vi "SPD.Update Lists.vi"(0 "SPD.Stand Ctrl in":T1 {"spdDeviceSession"."hidSPD.Controller"."HV_bias" format="%#_6p, V"; "spdDeviceSession"."hidSPD.Controller"."TSet" format="%#_6p, DegC"}, 11 "Error In":errorcluster, 12 "Temperature_List":refnum<vi>, 13 "Stb_code_List":refnum<vi>, 14 "HV_bias_List":refnum<vi>) -> (4 "SPD.Stand Ctrl out":T1 {"spdDeviceSession"."hidSPD.Controller"."HV_bias" format="%#_6p, V"; "spdDeviceSession"."hidSPD.Controller"."TSet" format="%#_6p, DegC"}, 15 "Error Out":errorcluster)   [LabVIEW 2018]
uses:
  typedefs/SPD.Stand Ctrl.ctl
  Instruments/SPD HID Interface/hidSPDLibForLabView/LibVIs/hidSPD Controls/hidSPD Device Session.ctl
  Instruments/SPD HID Interface/hidSPDLibForLabView/LibVIs/hidSPD Controls/hidSPD Controller.ctl
  Instruments/KC705 DevBoard/typedefs/DevB.Session.ctl
  Instruments/KeySight 53230A/typedefs/FreqC.Session.ctl
  Instruments/KeySight 8164B/KeySight 8164B LAN InstrLib/typedefs/KeySight 8164B control.ctl
  Instruments/LeCroy SDA830/typedefs/LeCroy.Session.ctl
  typedefs/SPD.Events.ctl
  <vilib>/Utility/config.llb/Config Data RefNum.ctl
  typedefs/SPD.Meas Result.ctl
  Instruments/SPD HID Interface/hidSPDLibForLabView/hidSPDLibForLabView.lvlib
  Instruments/KeySight 8164B/KeySight 8164B LAN InstrLib.lvlib
  <vilib>/Utility/config.llb/NI_LVConfig.lvlib
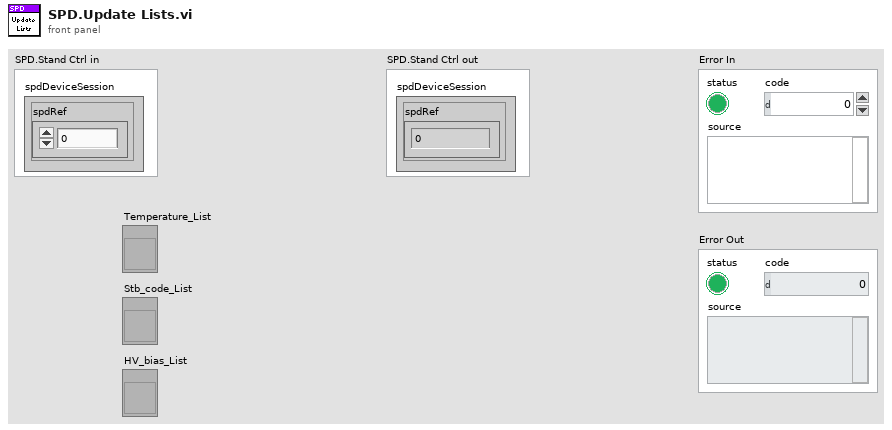
[diagram p1: front panel]
types:
  T1 = typedef "SPD.Stand Ctrl.ctl" = cluster{"spdDeviceSession":T2, "DevBSession":T4, "FreqCSession":T5, "8164BSession":T6, "LeCroySession":T7, "Events":T8, "configFile":T9, "SPD.Result":T10}
  T2 = typedef "hidSPDLibForLabView.lvlib/hidSPD Device Session.ctl" = cluster{"spdRef":u64, "connected":bool, "spdName":string, "hidSPD.Controller":T3}
  T3 = typedef "hidSPDLibForLabView.lvlib/hidSPD Controller.ctl" = cluster{"TSet":sgl, "HV_bias":sgl, "DDS_stb_code":u16}
  T4 = typedef "DevB.Session.ctl" = cluster{"DevBRef":refnum<visa-resource-name>, "connected":bool}
  T5 = typedef "FreqC.Session.ctl" = cluster{"FreqCRef":refnum<visa-resource-name>, "timeout":dbl, "Gate":dbl, "connected":bool}
  T6 = typedef "KeySight 8164B LAN InstrLib.lvlib/KeySight 8164B control.ctl" = cluster{"Connection ID":refnum<k5>, "Connected":bool, "Info":string, "Slots Info":string[]}
  T7 = typedef "LeCroy.Session.ctl" = cluster{"LeCroySession":refnum<visa-resource-name>, "connected":bool}
  T8 = typedef "SPD.Events.ctl" = cluster{"DCRTest":refnum<user-event>, "Stop":refnum<user-event>}
  T9 = typedef "NI_LVConfig.lvlib/Config Data RefNum.ctl" = refnum<k1>
  T10 = typedef "SPD.Meas Result.ctl" = cluster{"HV_Bias":dbl[][][], "Stb_code":dbl[], "Temprature":dbl[], "Data":dbl[][][][]}
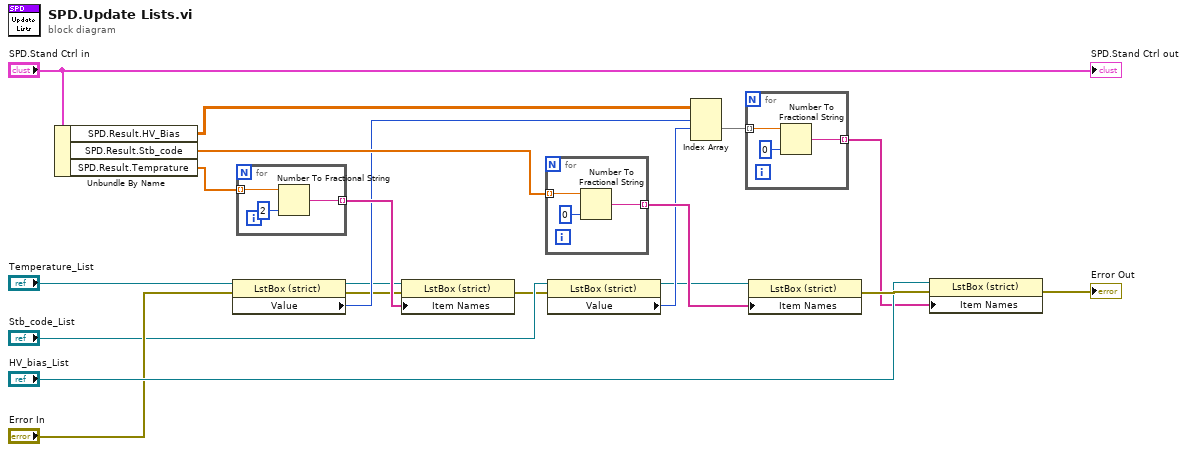
[diagram p0: block diagram]
diagram:
  n1 = Unbundle By Name("SPD.Stand Ctrl in") -> ("SPD.Result.HV_Bias"=w15:dbl[][][], "SPD.Result.Stb_code"=w17:dbl[], "SPD.Result.Temprature"=w20:dbl[])
  n2 = property class="LstBox (strict)"(reference="Temperature_List", error in="Error In") -> (reference out=w6:refnum<vi>, error out=w5:errorcluster, "Value"=w13:i32)
  n3 = for {
    tunnel: w20 -> [w23] mode=indexing
    tunnel: [w21] -> w18 mode=indexing
    n4 = Number To Fractional String(number=w23, precision (6)=i16 2) -> (F-format string=w21:string)  [unwired: 2 in]
  }
  n5 = property class="LstBox (strict)"(reference=w6, error in=w5, "Item Names"=w18) -> (error out=w3:errorcluster)  [unwired: 1 out]
  n6 = for {
    tunnel: w17 -> [w26] mode=indexing
    tunnel: [w24] -> w16 mode=indexing
    n7 = Number To Fractional String(number=w26, precision (6)=i16 0) -> (F-format string=w24:string)  [unwired: 2 in]
  }
  n8 = property class="LstBox (strict)"(reference="Stb_code_List", error in=w3) -> (reference out=w1:refnum<vi>, "Value"=w2:i32)  [unwired: 1 out]
  n9 = Index Array(array=w15, index (dim 0)=w13, index (dim 1)=w2) -> (element=w12:dbl[])  [unwired: 1 in]
  n10 = for {
    tunnel: [w28] -> w8 mode=indexing
    tunnel: w12 -> [w27] mode=indexing
    n11 = Number To Fractional String(number=w27, precision (6)=i16 0) -> (F-format string=w28:string)  [unwired: 2 in]
  }
  n12 = property class="LstBox (strict)"(reference=w1, "Item Names"=w16) -> (error out=w11:errorcluster)  [unwired: 1 in, 1 out]
  n13 = property class="LstBox (strict)"(reference="HV_bias_List", error in=w11, "Item Names"=w8) -> (error out=→"Error Out":errorcluster)  [unwired: 1 out]
  "SPD.Stand Ctrl out" <- "SPD.Stand Ctrl in"
